vi "WPI_IMU_ADIS16448_Get Instant.vi"(8 "error in":errorcluster, 11 "ADI IMU Interrupt DevRef":T2={"ADI IMU DevRef"={"DevStatus"={"status"=FALSE, "code"=0, "source"=""}, "Handle"=0, "SPI Bus"=enum."SPI On-Board, CS0", "Device Found"=FALSE, "Device Ready"=FALSE, "Yaw Axis"=enum."Z", "AHRS Algorithm"=enum."Complementary", "Serial"=0, "Lot ID 2"=0, "Lot ID 1"=0, "Product ID"=0}, "InterruptRef"={"DevStatus"={"status"=FALSE, "code"=0, "source"=""}, "InterruptIndex"=enum."0"}}) -> (0 "error out":errorcluster, 1 "Sensor Ready Out":bool, 2 "IMU Data Out":T1, 3 "ADI IMU Interrupt DevRef Out":T2={"ADI IMU DevRef"={"DevStatus"={"status"=FALSE, "code"=0, "source"=""}, "Handle"=0, "SPI Bus"=enum."SPI On-Board, CS0", "Device Found"=FALSE, "Device Ready"=FALSE, "Yaw Axis"=enum."Z", "AHRS Algorithm"=enum."Complementary", "Serial"=0, "Lot ID 2"=0, "Lot ID 1"=0, "Product ID"=0}, "InterruptRef"={"DevStatus"={"status"=FALSE, "code"=0, "source"=""}, "InterruptIndex"=enum."0"}})   [LabVIEW 2015, in "Apple Pi Gyro Library.lvlib" / "FRC_ADIS16448_IMU.lvlib"]
doc: "Get instantaneous readings from the Analog Devices MXP IMU board (Gyro Rate, Accel, Magnetometer, Barometer, Temp). This requires that the IMU_Loop VI be located in Periodic Tasks."
uses:
  FRC_ADIS16448_IMU.lvlib
  WPI_IMU_ADIS16448_InterruptDevRef.ctl
  WPI_IMU_ADIS16448_IMUDevRef.ctl
  <vilib>/Rock Robotics/SystemInterfaces/spilib/spi_bus.ctl
  <vilib>/Rock Robotics/WPI/Interrupt/WPI_InterruptRef.ctl
  <vilib>/Rock Robotics/SystemInterfaces/Interrupt/FPGA_InterruptIndex.ctl
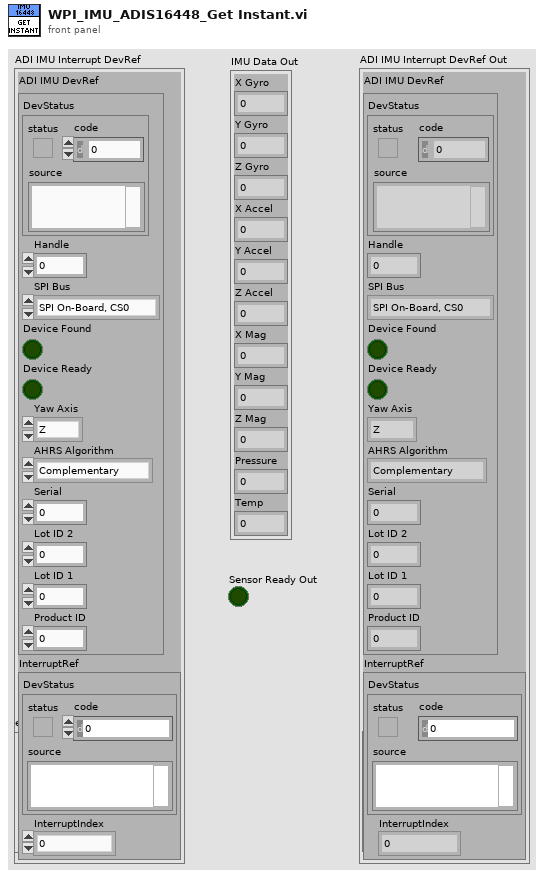
[diagram p1: front panel]
types:
  T1 = cluster{"X Gyro":dbl, "Y Gyro":dbl, "Z Gyro":dbl, "X Accel":dbl, "Y Accel":dbl, "Z Accel":dbl, "X Mag":dbl, "Y Mag":dbl, "Z Mag":dbl, "Pressure":dbl, "Temp":dbl}
  T2 = typedef "Apple Pi Gyro Library.lvlib/FRC_ADIS16448_IMU.lvlib/WPI_IMU_ADIS16448_InterruptDevRef.ctl" = cluster{"ADI IMU DevRef":T3, "InterruptRef":T5}
  T3 = typedef "Apple Pi Gyro Library.lvlib/FRC_ADIS16448_IMU.lvlib/WPI_IMU_ADIS16448_IMUDevRef.ctl" = cluster{"DevStatus":errorcluster, "Handle":i32, "SPI Bus":T4, "Device Found":bool, "Device Ready":bool, "Yaw Axis":enum16{"X", "Y", "Z"}, "AHRS Algorithm":enum16{"Complementary", "Madgwick"}, "Serial":u16, "Lot ID 2":u16, "Lot ID 1":u16, "Product ID":u16}
  T4 = typedef "spi_bus.ctl" = enum16{"SPI On-Board, CS0", "SPI On-Board, CS1", "SPI On-Board, CS2", "SPI On-Board, CS3", "SPI MXP", "Invalid"}
  T5 = typedef "WPI_InterruptRef.ctl" = cluster{"DevStatus":errorcluster, "InterruptIndex":T6}
  T6 = typedef "FPGA_InterruptIndex.ctl" = enum8{"0", "1", "2", "3", "4", "5", "6", "7", "Invalid"}
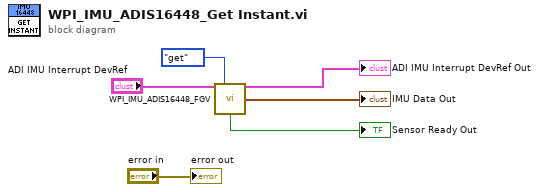
[diagram p0: block diagram]
diagram:
  n1 = call "WPI_IMU_ADIS16448_FGV.vi"("ADI IMU Interrupt DevRef"="ADI IMU Interrupt DevRef", "Operation"=enum16{"set", "get", "set reset"}."get") -> ("ADI IMU Interrupt DevRef Out"=→"ADI IMU Interrupt DevRef Out":T2, "IMU Data Out"=→"IMU Data Out":T1, "Sensor Ready Out"=→"Sensor Ready Out":bool)  [unwired: 7 in, 4 out]
  "error out" <- "error in"
